vi "ManipWaitForArm.vi"(2 "Reinit":bool, 3 "Parameter String":string) -> (0 "error out":errorcluster, 1 "Advance Trigger":bool)   [LabVIEW 2020]
doc: "This VI requires the maniplator sequencer to wait until the arm has reached its goal position.\n\nParameters:\nNone"
uses:
  SafeParser_String.vi
  GlobalArm.vi
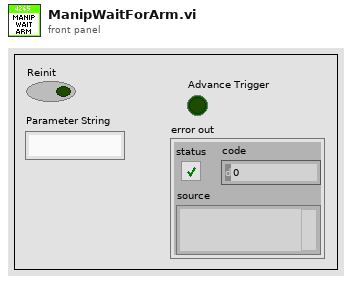
[diagram p1: front panel]
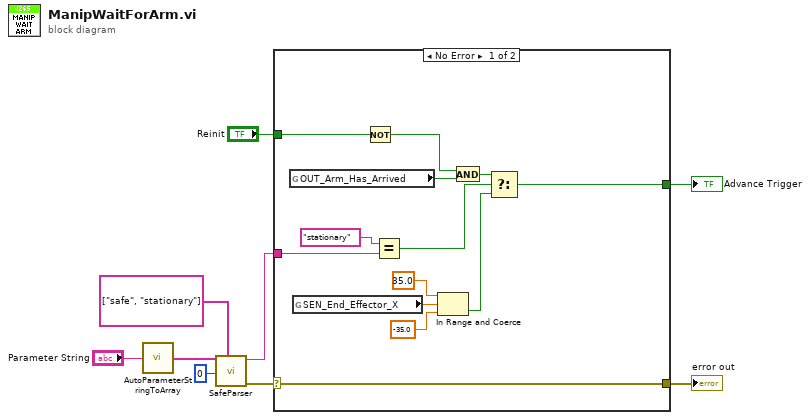
[diagram p0: block diagram]
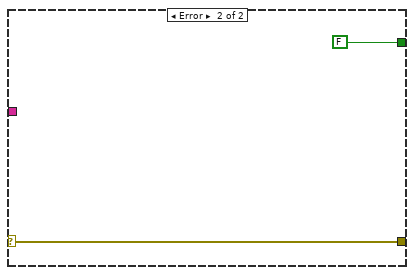
[diagram p2: hidden frame]
diagram:
  n1 = call "AutoParameterStringToArray.vi"("Parameter String"="Parameter String") -> ("Parsed Parameters"=w6:string[])
  n2 = call-poly "SafeParser.vi"("Allowed Values"=string[] ["safe", "stationary"], "Array Index"=0 ("Parameter Index"), "String Array"=w6) -> ("Error Out"=w3:errorcluster, "Typecast Value"=w2:string)  [unwired: 7 in]
  n3 = case shown="No Error" w3 {
    selector: w3 -> [w22 w23]
    tunnel: [w13 FALSE] -> w9
    tunnel: [w22 w23] -> w4
    tunnel: w2 -> [w21 _]
    tunnel: "Reinit" -> [w11 _]
    frame No Error {
      n4 = global read "GlobalArm.vi" "OUT_Arm_Has_Arrived"() -> (w14:bool)
      n5 = global read "GlobalArm.vi" "SEN_End_Effector_X"() -> (w18:dbl)
      n6 = Not(x=w11) -> (.not. x?=w10:bool)
      n7 = Equal?(x="stationary", y=w21) -> (x = y?=w19:bool)
      n8 = In Range and Coerce(upper limit=35.0, x=w18, lower limit=-35.0) -> (In Range?=w15:bool)  [unwired: 1 out]
      n9 = And(x=w10, y=w14) -> (x .and. y?=w12:bool)
      n10 = Select(t=w12, s=w19, f=w15) -> (s? t:f=w13:bool)
    }
    frame Error {
    }
  }
  "Advance Trigger" <- w9
  "error out" <- w4
